vi "Parse Labels in Channel.vi"(8 "error in":errorcluster, 9 "channel #":u16, 10 "direction":T1, 11 "node in":refnum<k20>) -> (0 "error out":errorcluster, 3 "labels":T2[](array[typedef]))   [LabVIEW 2024, in "ARINC 429 Import.lvlib"]
uses:
  ARINC 429 Import.lvlib
  Shared/VS Channels Definition for Label.ctl
  Shared/VS Channel Definition for Parameter.ctl
  Shared/Parameter Definition.ctl
  <vilib>/NI/NI VeriStand Encoding and Decoding/Encoding.ctl
  Shared/Transfer Type.ctl
  Shared/Direction.ctl
  Shared/Error Word Bits Checker.vi
  Read Tag Element (U16).vi
  Read Tag Element (U32).vi
  Read Tag Element (String).vi
  Read Tag Element (Boolean).vi
  <vilib>/NI/NI VeriStand Encoding and Decoding/Encoding and Decoding.lvlib
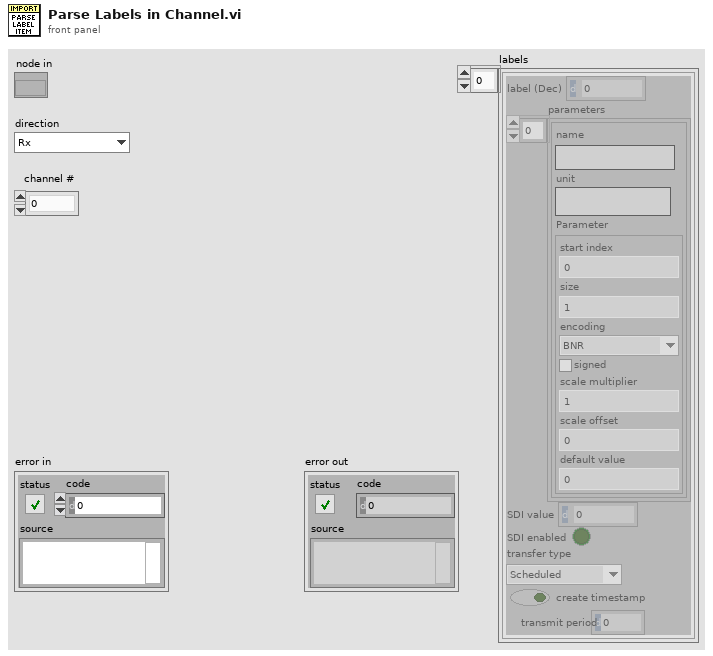
[diagram p1: front panel]
types:
  T1 = typedef "Direction.ctl" = enum16{"Rx", "Tx"}
  T2 = typedef "VS Channels Definition for Label.ctl" = cluster{"label (Dec)":u32, "parameters":T3[], "SDI value":u8, "SDI enabled":bool, "transfer type":T6, "create timestamp":bool, "transmit period":u32}
  T3 = typedef "VS Channel Definition for Parameter.ctl" = cluster{"name":string, "unit":string, "Parameter":T4}
  T4 = typedef "Parameter Definition.ctl" = cluster{"start index":i32, "size":i32, "encoding":T5, "signed":bool, "scale multiplier":dbl, "scale offset":dbl, "default value":dbl}
  T5 = typedef "Encoding and Decoding.lvlib/Encoding.ctl" = enum16{"BNR", "BCD", "Discrete"}
  T6 = typedef "Transfer Type.ctl" = enum16{"Scheduled", "Acyclic", "Block", "Strobe"}
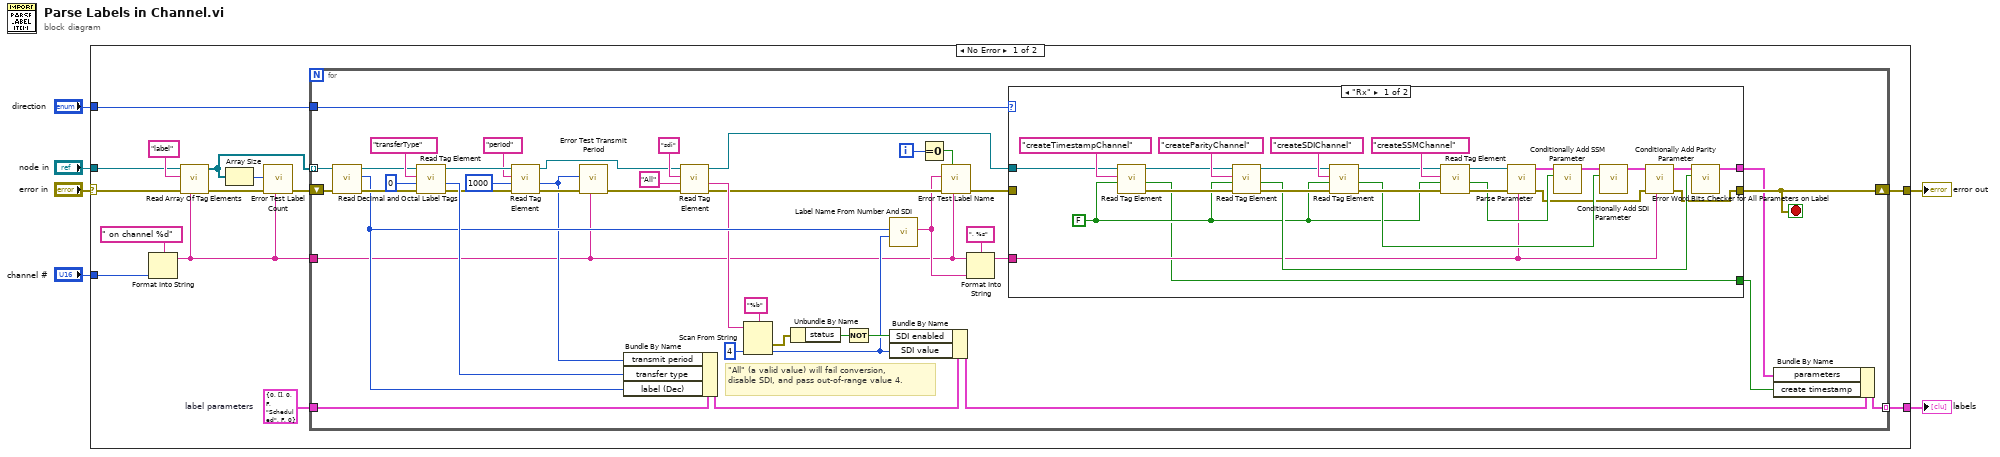
[diagram p0: block diagram]
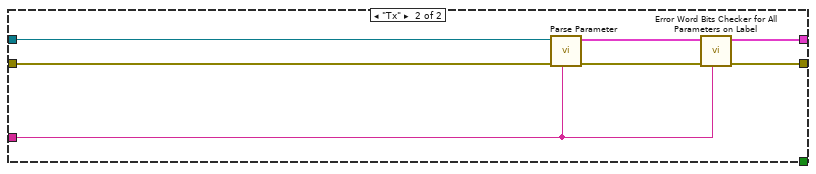
[diagram p2: hidden frame]
diagram:
  n1 = case shown="No Error" "error in" {
    selector: "error in" -> [w13 w96]
    tunnel: [w20 _] -> w6
    tunnel: "node in" -> [w16 _]
    tunnel: [w15 w96] -> w4
    tunnel: "direction" -> [w14 _]
    tunnel: "channel #" -> [w9 _]
    frame No Error {
      w11 = T2 {"label (Dec)"=0, "parameters"=[], "SDI value"=0, "SDI enabled"=FALSE, "transfer type"=enum."Scheduled", "create timestamp"=FALSE, "transmit period"=0}  # label parameters
      n2 = Format Into String(format string=" on channel %d", w9) -> (resulting string=w10:string)  [unwired: 2 in, 1 out]
      n3 = call "Read Array Of Tag Elements.vi"("error text in"=w10, "error in"=w13, "tag name"="label" ("Tag Name"), "node in"=w16) -> ("error out"=w18:errorcluster, "array of elements"=w7:refnum<k20>[])  [unwired: 6 in]
      n4 = Array Size(array=w7) -> (size(s)=w8:i32)
      n5 = call "Error Test Label Count.vi"("error text in"=w10, "error in"=w18, "number of labels"=w8) -> ("error out"=w17:errorcluster)  [unwired: 8 in]
      n6 = for {
        shift-right: [w42] -> w15
        shift-left: w17 -> [w45]
        tunnel: [w54] -> w20 mode=indexing
        tunnel: w7 -> [w52] mode=indexing
        tunnel: w14 -> [w43]
        tunnel: w11 -> [w46]
        tunnel: w10 -> [w22]
        i -> [w34]
        stop <- w42 stop-if-true
        # "\"All\" (a valid value) will fail conversion, disable SDI, and pass out-of-range value 4."
        n7 = call "Read Decimal and Octal Label Tags.vi"("error in"=w45, "node in"=w52) -> ("error out"=w49:errorcluster, "label (Dec)"=w39:u32, "node out"=w50:refnum<k20>)  [unwired: 7 in]
        n8 = call-poly "Read Tag Element.vi"("error in"=w49, "default"=u16 0, "Tag Name"="transferType", "node in"=w50) -> ("error out"=w28:errorcluster, "value"=w47:u16, "node out"=w29:refnum<k20>)  [unwired: 5 in]
        n9 = call-poly "Read Tag Element.vi"("error in"=w28, "default"=u32 1000, "Tag Name"="period", "node in"=w29) -> ("error out"=w25:errorcluster, "value"=w23:u32, "node out"=w21:refnum<k20>)  [unwired: 5 in]
        n10 = call "Error Test Transmit Period.vi"("error text in"=w22, "error in"=w25, "transmit period"=w23) -> ("error out"=w24:errorcluster)  [unwired: 8 in]
        n11 = Bundle By Name(cluster=w46, "transmit period"=w23, "transfer type"=w47, "label (Dec)"=w39) -> (w53:T2)
        n12 = call-poly "Read Tag Element.vi"("error in"=w24, "default"="All", "Tag Name"="sdi", "node in"=w21) -> ("error out"=w37:errorcluster, "value"=w38:string, "node out"=w35:refnum<k20>)  [unwired: 5 in]
        n13 = Scan From String(format string="%b", input string=w38, default 1=u8 4 ("default value 1")) -> (error out=w58:errorcluster, output 1=w31:u8)  [unwired: 2 in, 2 out]
        n14 = Unbundle By Name(w58) -> ("status"=w57:bool)
        n15 = Not(x=w57) -> (.not. x?=w56:bool)
        n16 = call "Label Name From Number And SDI.vi"("SDI value"=w31, "label (Dec)"=w39) -> ("label name"=w32:string)  [unwired: 9 in]
        n17 = Bundle By Name(cluster=w53, "SDI enabled"=w56, "SDI value"=w31) -> (w55:T2)
        n18 = Equal To 0?(x=w34) -> (x = 0?=w33:bool)
        n19 = call "Error Test Label Name.vi"("error text in"=w22, "reset (F)"=w33, "error in"=w37, "label name"=w32) -> ("error out"=w36:errorcluster)  [unwired: 7 in]
        n20 = Format Into String(format string=", %s", initial string=w22, w32) -> (resulting string=w41:string)  [unwired: 1 in, 1 out]
        n21 = case shown="\"Rx\"" w43 {
          tunnel: [w70 w94] -> w42
          tunnel: w41 -> [w69 w89]
          tunnel: [w81 w93] -> w40
          tunnel: w35 -> [w67 w92]
          tunnel: w36 -> [_ w91]
          tunnel: [w63 _] -> w30
          frame "Rx" {
            w64 = FALSE
            n22 = call-poly "Read Tag Element.vi"("default"=w64, "Tag Name"="createTimestampChannel", "node in"=w67) -> ("error out"=w65:errorcluster, "value"=w63:bool, "node out"=w66:refnum<k20>)  [unwired: 6 in]
            n23 = call-poly "Read Tag Element.vi"("error in"=w65, "default"=w64, "Tag Name"="createParityChannel", "node in"=w66) -> ("error out"=w79:errorcluster, "value"=w73:bool, "node out"=w80:refnum<k20>)  [unwired: 5 in]
            n24 = call-poly "Read Tag Element.vi"("error in"=w79, "default"=w64, "Tag Name"="createSDIChannel", "node in"=w80) -> ("error out"=w84:errorcluster, "value"=w83:bool, "node out"=w85:refnum<k20>)  [unwired: 5 in]
            n25 = call-poly "Read Tag Element.vi"("error in"=w84, "default"=w64, "Tag Name"="createSSMChannel", "node in"=w85) -> ("error out"=w77:errorcluster, "value"=w72:bool, "node out"=w78:refnum<k20>)  [unwired: 5 in]
            n26 = call "Parse Parameter.vi"("error text in"=w69, "error in"=w77, "node in"=w78) -> ("error out"=w71:errorcluster, "parametesrs"=w76:T3[])  [unwired: 7 in]
            n27 = call "Conditionally Add SSM Parameter.vi"("create SSM (F)"=w72, "parameters in"=w76) -> ("parameters out"=w75:T3[])  [unwired: 9 in]
            n28 = call "Conditionally Add SDI Parameter.vi"("create SDI (F)"=w83, "parameters in"=w75) -> ("parameters out"=w74:T3[])  [unwired: 9 in]
            n29 = call "Error Word Bits Checker for All Parameters on Label.vi"("error text in"=w69, "error in"=w71, "parameters in"=w74) -> ("error out"=w70:errorcluster, "parameters out"=w82:T3[])  [unwired: 7 in]
            n30 = call "Conditionally Add Parity Parameter.vi"("create parity (F)"=w73, "parameters in"=w82) -> ("parameters out"=w81:T3[])  [unwired: 9 in]
          }
          frame "Tx" {
            n31 = call "Parse Parameter.vi"("error text in"=w89, "error in"=w91, "node in"=w92) -> ("error out"=w95:errorcluster, "parametesrs"=w90:T3[])  [unwired: 7 in]
            n32 = call "Error Word Bits Checker for All Parameters on Label.vi"("error text in"=w89, "error in"=w95, "parameters in"=w90) -> ("error out"=w94:errorcluster, "parameters out"=w93:T3[])  [unwired: 7 in]
          }
        }
        n33 = Bundle By Name(cluster=w55, "parameters"=w40, "create timestamp"=w30) -> (w54:T2)
      }
    }
    frame Error {
    }
  }
  "labels" <- w6
  "error out" <- w4
